vi "Deform_Mirror_VMap_ae.vi"(1 "Action":enum16{"WRITE", "READ"}(ring), 7 "V Map In":dbl[][](array[numeric])) -> (8 "V Map Out":dbl[][](array[numeric]))   [LabVIEW 2014]
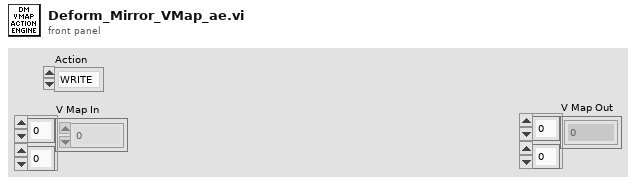
[diagram p1: front panel]
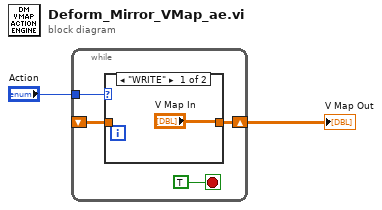
[diagram p0: block diagram]
diagram:
  n1 = while {
    tunnel: "Action" -> [w5]
    shift-right: [w3] -> w1
    shift-left: _ -> [w4]
    stop <- TRUE stop-if-true
    n2 = case shown="\"WRITE\"" w5 {
      tunnel: w4 -> [_ w8]
      tunnel: ["V Map In" w8] -> w3
      frame "WRITE" {
      }
      frame "READ" {
      }
    }
  }
  "V Map Out" <- w1
